vi "Get registry path.vi"() -> (3 "Registry path":path)   [LabVIEW 2014]
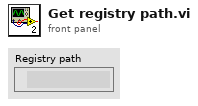
[diagram p1: front panel]
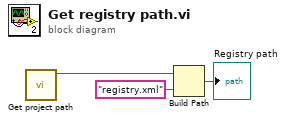
[diagram p0: block diagram]
diagram:
  n1 = call "Get project path.vi"() -> ("Project path"=w2:path)  [unwired: 11 in]
  n2 = Build Path(base path=w2, name or relative path="registry.xml") -> (appended path=→"Registry path":path)
